vi "ZPK_2_TF.vi"(8 "error in (no error)":errorcluster, 11 "ZPK model":T2) -> (0 "error out":errorcluster, 3 "TF model":T1 {"Denominator" format="%#.15g"; "Numerator" format="%#.15g"})   [LabVIEW 2020, in "PC-RT_Controller.lvlib"]
doc: "Convert ZPK model into TF model."
uses:
  PC-RT_Controller.lvlib
  TypeDefs/ZPK_model.ctl
  TypeDefs/TF_model.ctl
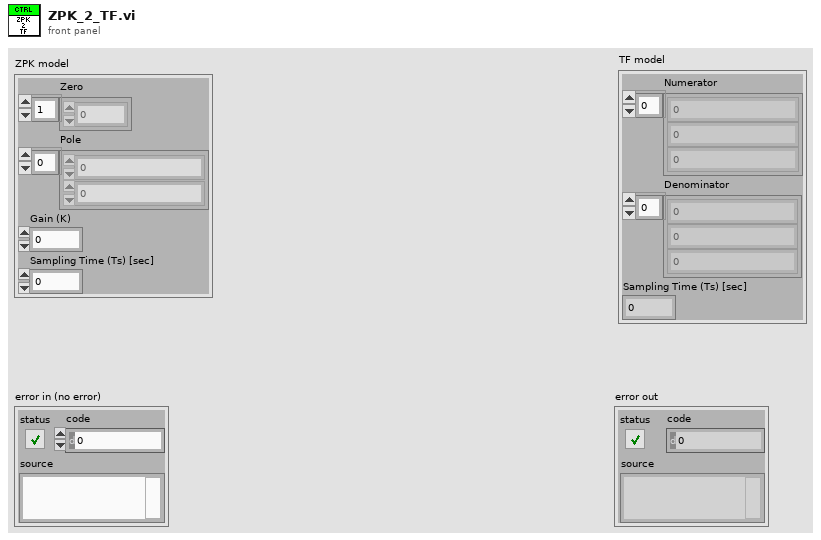
[diagram p1: front panel]
types:
  T1 = typedef "PC-RT_Controller.lvlib/TF_model.ctl" = cluster{"Numerator":dbl[], "Denominator":dbl[], "Sampling Time (Ts) [sec]":dbl}
  T2 = typedef "PC-RT_Controller.lvlib/ZPK_model.ctl" = cluster{"Zero":cdb[], "Pole":cdb[], "Gain (K)":dbl, "Sampling Time (Ts) [sec]":dbl}
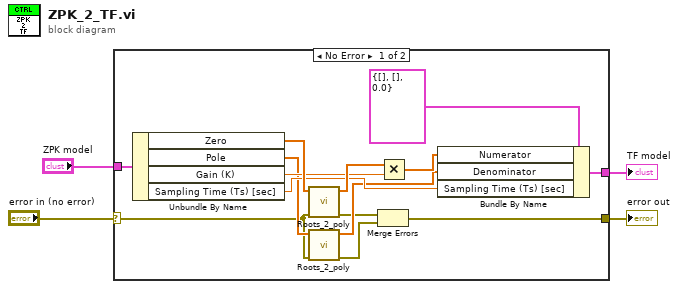
[diagram p0: block diagram]
diagram:
  n1 = case shown="No Error" "error in (no error)" {
    selector: "error in (no error)" -> [w8 w19]
    tunnel: [w7 w19] -> w3
    tunnel: "ZPK model" -> [w18 _]
    tunnel: [w9 _] -> w1
    frame No Error {
      n2 = Unbundle By Name(w18) -> ("Zero"=w17:cdb[], "Pole"=w11:cdb[], "Gain (K)"=w15:dbl, "Sampling Time (Ts) [sec]"=w13:dbl)
      n3 = call "Roots_2_poly.vi"("error in (no error)"=w8, "Roots"=w17) -> ("error out"=w6:errorcluster, "Polynomial Coeffcients"=w16:dbl[])  [unwired: 8 in]
      n4 = call "Roots_2_poly.vi"("error in (no error)"=w8, "Roots"=w11) -> ("error out"=w5:errorcluster, "Polynomial Coeffcients"=w10:dbl[])  [unwired: 8 in]
      n5 = Merge Errors(w6, w5) -> (w7:errorcluster)
      n6 = Multiply(x=w16, y=w15) -> (x*y=w12:dbl[])
      n7 = Bundle By Name(cluster=T1 {"Numerator"=[], "Denominator"=[], "Sampling Time (Ts) [sec]"=0.0} ("TF model"), "Numerator"=w12, "Denominator"=w10, "Sampling Time (Ts) [sec]"=w13) -> (w9:T1)
    }
    frame Error {
    }
  }
  "error out" <- w3
  "TF model" <- w1
